vi "Get Metadata.vi"(8 "error in (no error)":errorcluster, 11 "session id in":i32) -> (0 "error out":errorcluster, 2 "Metadata":string[][](table), 3 "session id out":i32)   [LabVIEW 2017, in "libonnx_wrapper.lvlib"]
doc: "Get Metadata from ONNX"
uses:
  libonnx_wrapper.lvlib
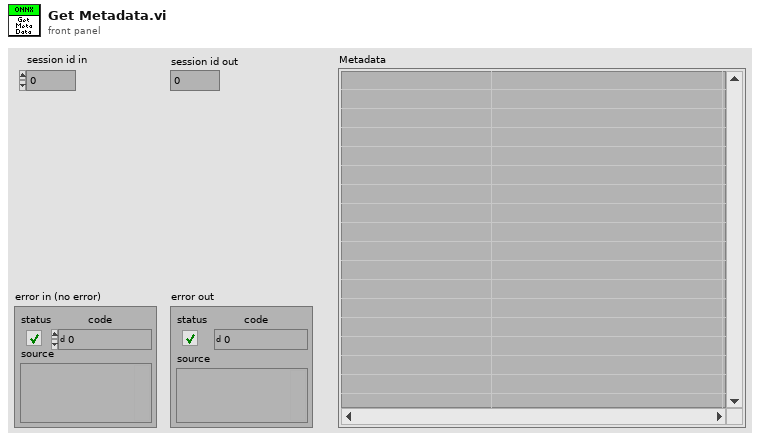
[diagram p1: front panel]
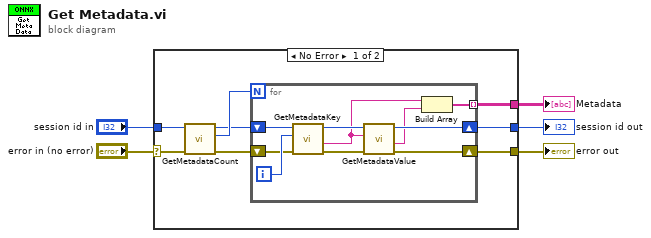
[diagram p0: block diagram]
diagram:
  n1 = case shown="No Error" "error in (no error)" {
    selector: "error in (no error)" -> [w6 w24]
    tunnel: [w10 _] -> w5
    tunnel: [w9 w24] -> w4
    tunnel: "session id in" -> [w8 w25]
    tunnel: [w7 w25] -> w2
    frame No Error {
      n2 = call "GetMetadataCount.vi"("error in (no error)"=w6, "session id in"=w8) -> ("error out"=w11:errorcluster, "MetadataCount"=w13:i32, "session id out"=w12:i32)  [unwired: 7 in]
      n3 = for {
        N: w13 -> [_]
        shift-right: [w18] -> w7
        shift-left: w12 -> [w23]
        shift-right: [w17] -> w9
        shift-left: w11 -> [w21]
        tunnel: [w14] -> w10 mode=indexing
        i -> [w22]
        n4 = call "GetMetadataKey.vi"("error in (no error)"=w21, "index"=w22, "session id in"=w23) -> ("error out"=w19:errorcluster, "MetadataKey"=w16:string, "session id out"=w20:i32)  [unwired: 6 in]
        n5 = call "GetMetadataValue.vi"("error in (no error)"=w19, "key"=w16, "session id in"=w20) -> ("error out"=w17:errorcluster, "MetadataValue"=w15:string, "session id out"=w18:i32)  [unwired: 6 in]
        n6 = Build Array(w16, w15) -> (w14:string[])
      }
    }
    frame Error {
    }
  }
  "Metadata" <- w5
  "error out" <- w4
  "session id out" <- w2
